vi "GetTextplain.vi"(8 "error in (no error)":errorcluster, 11 "object in":refnum<class "execute_result Message.lvclass">) -> (0 "error out":errorcluster, 2 "text/plain":string, 3 "object out":refnum<class "execute_result Message.lvclass">)   [LabVIEW 2018]
uses:
  execute_result Message.lvclass
  C:/Users/gavin/Documents/LabVIEW Data/LabVIEW-Bits/Connectivity/Jupyter Client/IOPub Messages/display_data Message/display_data Message.lvclass
  C:/Users/gavin/Documents/LabVIEW Data/LabVIEW-Bits/Connectivity/Jupyter Client/Base Classes/Message Class/Message Class.lvclass
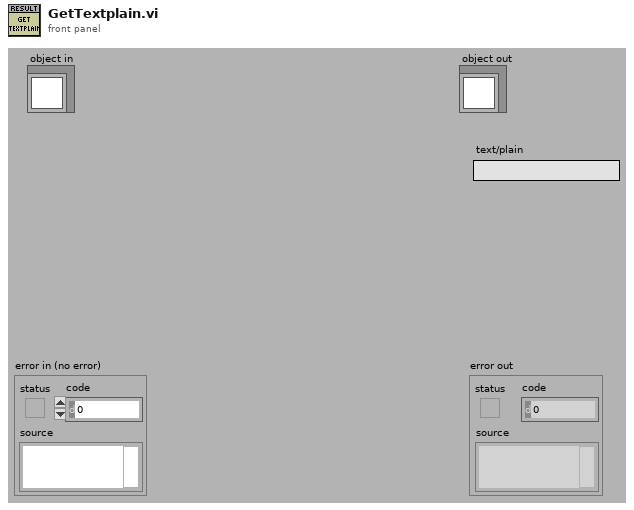
[diagram p1: front panel]
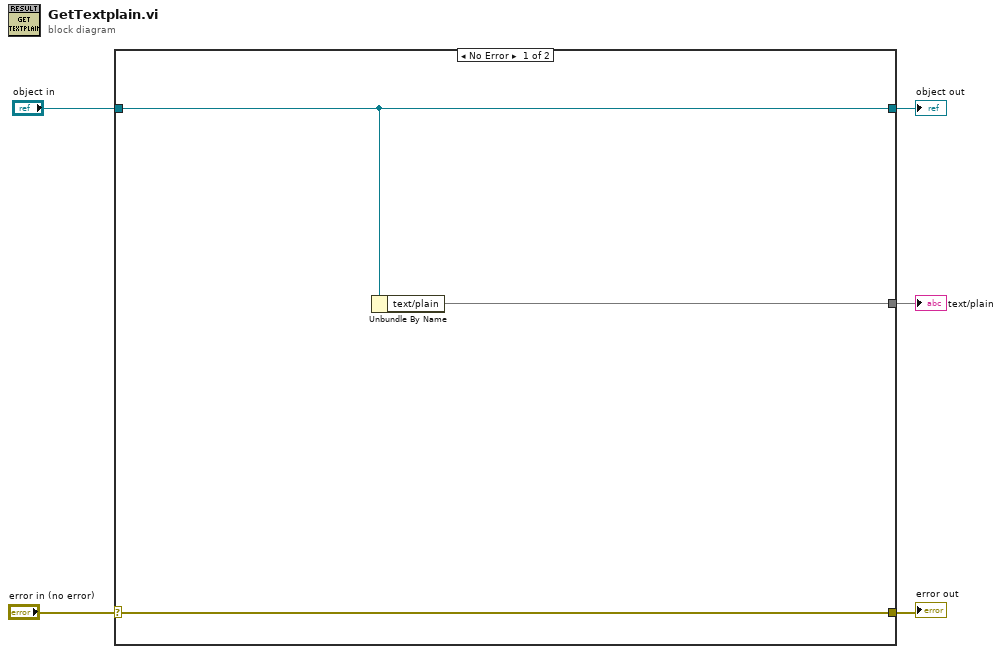
[diagram p0: block diagram]
diagram:
  n1 = case shown="No Error" "error in (no error)" {
    selector: "error in (no error)" -> [w7 w10]
    tunnel: [w7 w10] -> w4
    tunnel: [w6 w9] -> w2
    tunnel: "object in" -> [w6 w9]
    tunnel: [w8 _] -> w1
    frame No Error {
      n2 = Unbundle By Name(w6) -> ("text/plain"=w8)
    }
    frame Error {
    }
  }
  "error out" <- w4
  "object out" <- w2
  "text/plain" <- w1
